vi "_deleteme.vi"() -> ()   [LabVIEW 2016, in "SMD-7615.lvlib"]
uses:
  SMD-7615.lvlib
  <resource>/objmgr/nimcca.rc
panel:
  out "error out":errorcluster
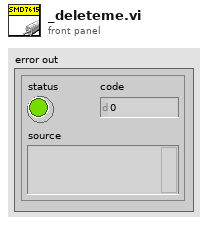
[diagram p1: front panel]
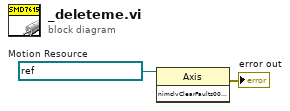
[diagram p0: block diagram]
diagram:
  w2 = refnum<k21> "niss:\\\\192.168.1.10"  # Motion Resource
  n1 = invoke class="Axis" method="nimclvClearFaults00A10001"(reference=w2) -> (error out=→"error out":errorcluster)  [unwired: 2 in, 2 out]
